vi "Axsun control.vi"() -> ()   [LabVIEW 2018]
uses:
  General/Controls/QueueNames.ctl
  General/Controls/Queue Manager Actions.ctl
  General/Controls/MessagePacket.ctl
  C:/Users/shuaibin/Documents/SerialSectOCT/SerialSectOCT/Software/Test Code/Stephan/Axsun Control/AxsunOCTControl.dll
  AxsunOCTControl.dll
panel:
  out "Cluster":cluster{i32, string[], string, dbl, string, i32}
  out "GUI error":errorcluster
  in  "Source current OFF":bool
  in  "Source current ON":bool
  in  "stop":bool
  in  "Laser OFF":bool
  in  "Laser ON":bool
  out "processor error":errorcluster
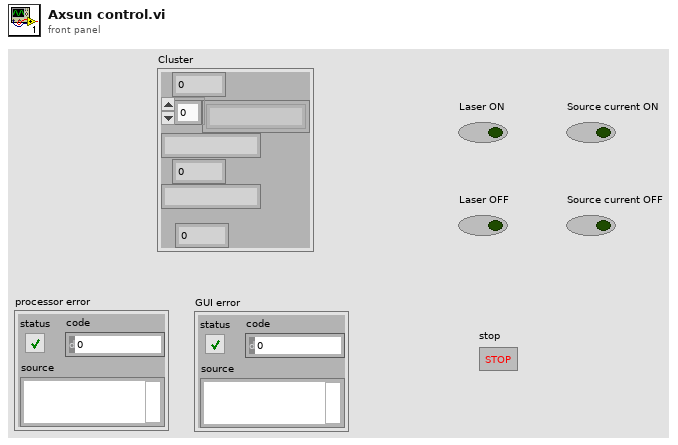
[diagram p1: front panel]
types:
  T1 = typedef "MessagePacket.ctl" = cluster{"Message":string, "Parameter":variant}
  T2 = typedef "Queue Manager Actions.ctl" = enum16{"Init", "Enqueue", "Enqueue All", "Preview Queue", "Dequeue", "Get Status", "Flush Queue", "Flush All Queues", "Release All Queues", "Release Queue", "Enqueue at Opposite End"}
  T3 = typedef "QueueNames.ctl" = enum16{"Main GUI", "Main Scan Processor", "Axsun GUI", "Axsun processor", "Main Display", "Main Table Stage GUI", "Main Table Stage Proc.", "Scan Engine", "Vibratome GUI", "Vibratome Processor", "Slice Engine"}
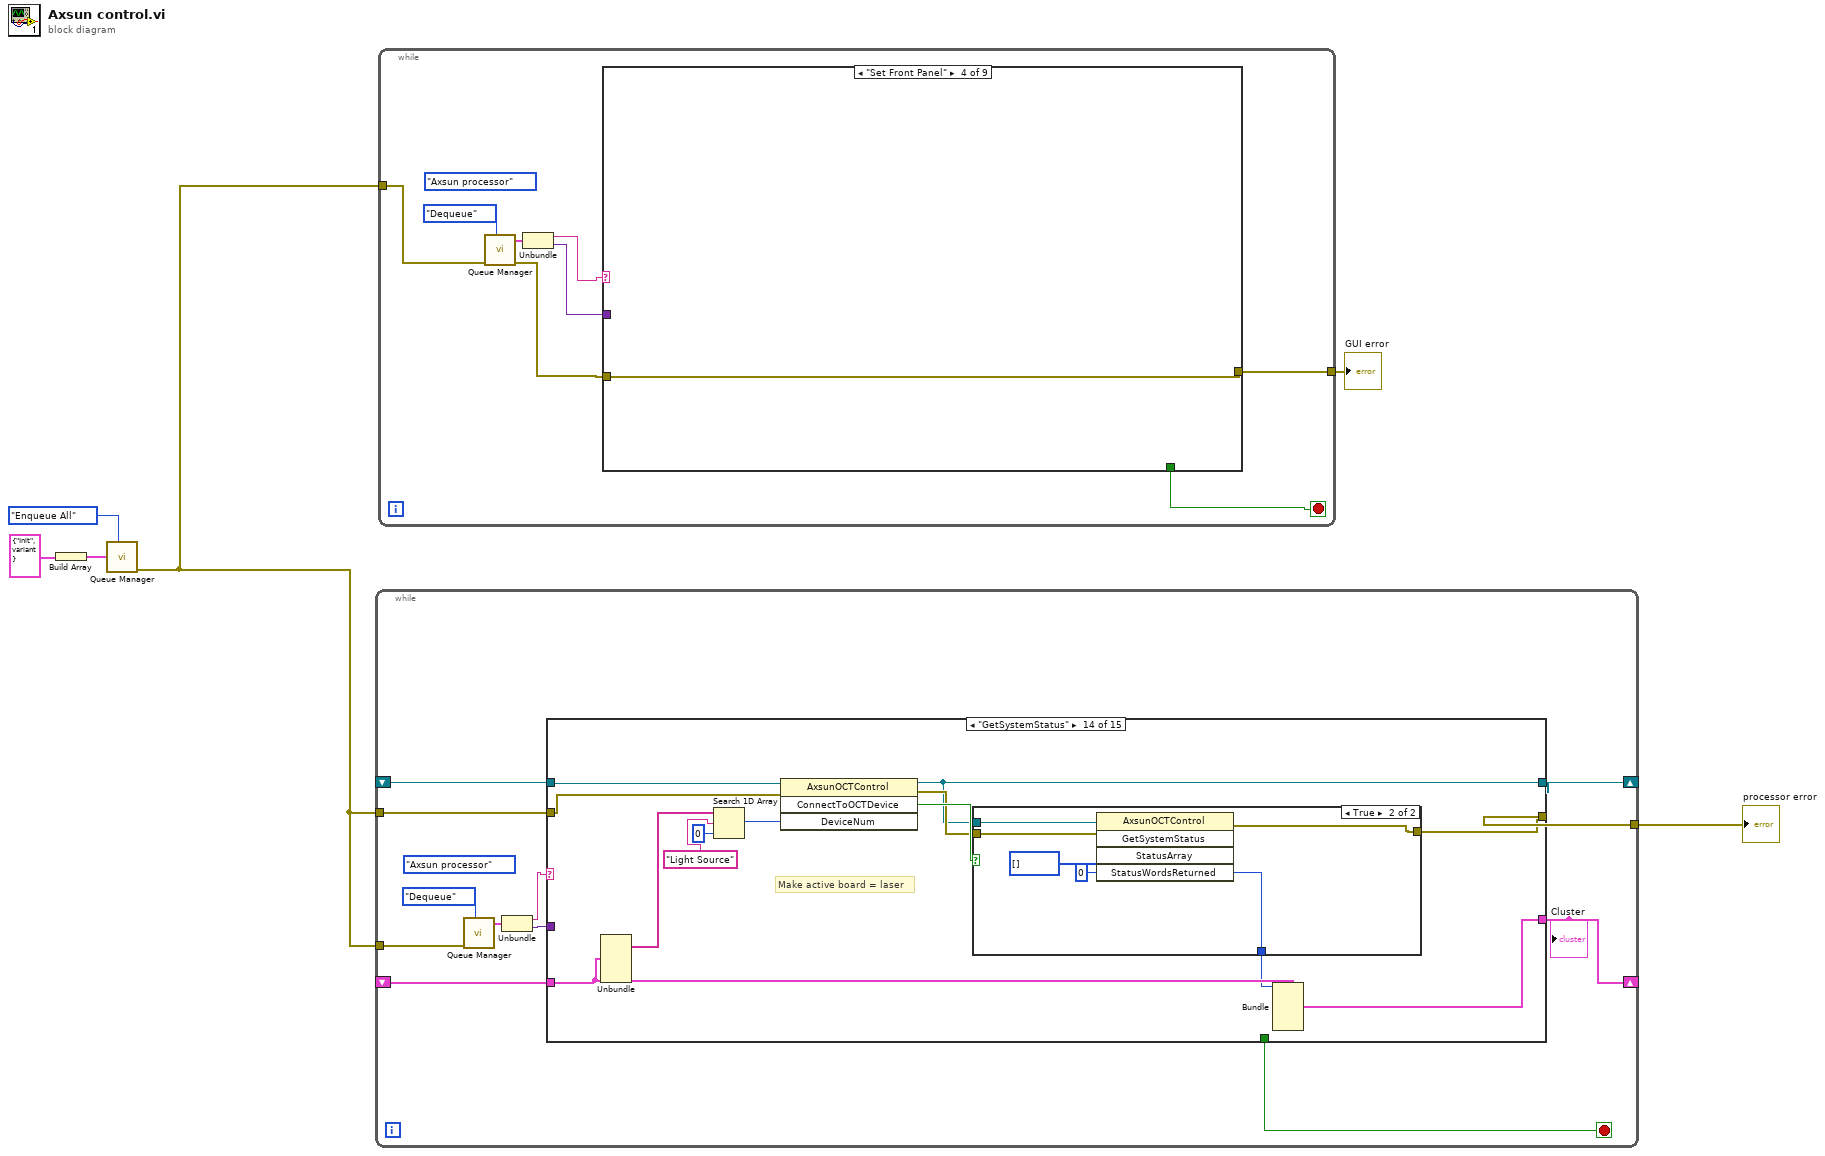
[diagram p0: block diagram]
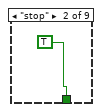
[diagram p3: hidden frame]
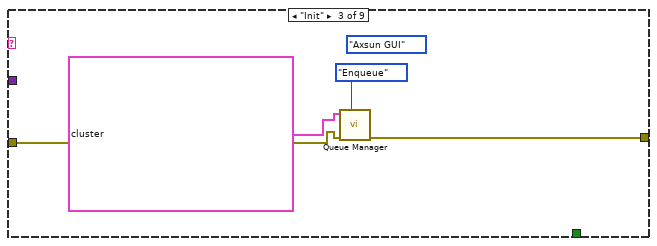
[diagram p4: hidden frame]
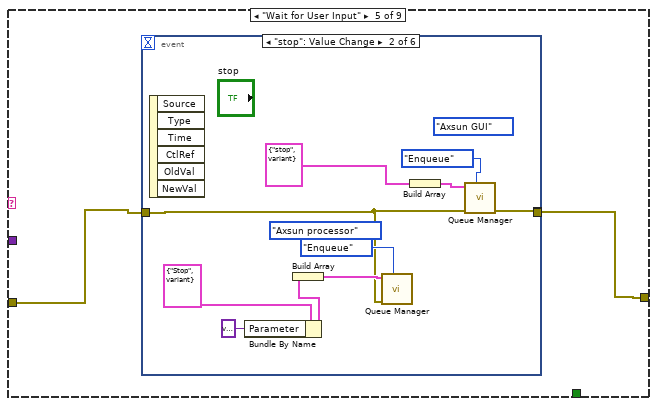
[diagram p5: hidden frame]
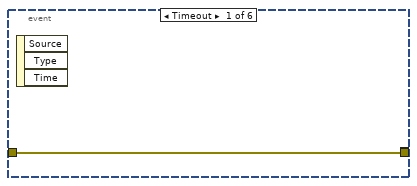
[diagram p6: hidden frame]
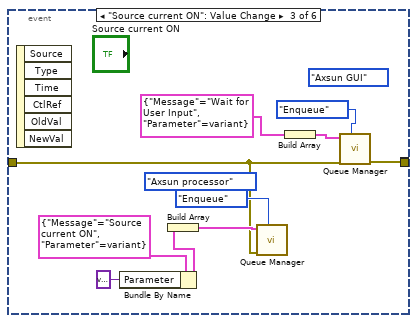
[diagram p7: hidden frame]
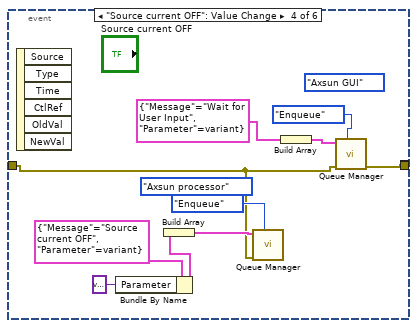
[diagram p8: hidden frame]
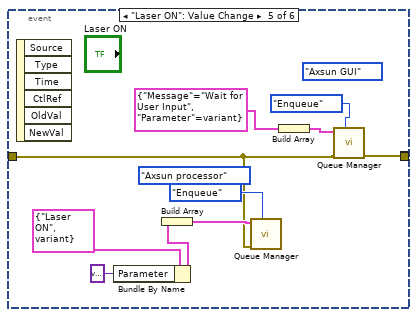
[diagram p9: hidden frame]
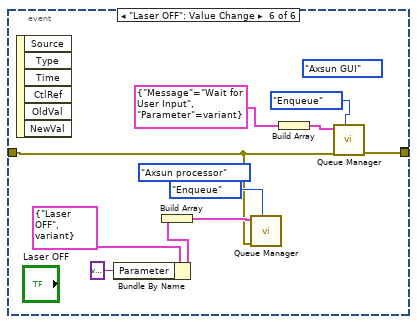
[diagram p10: hidden frame]
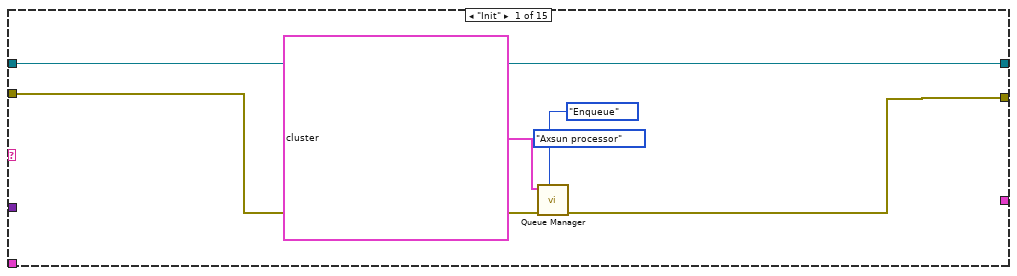
[diagram p15: hidden frame]
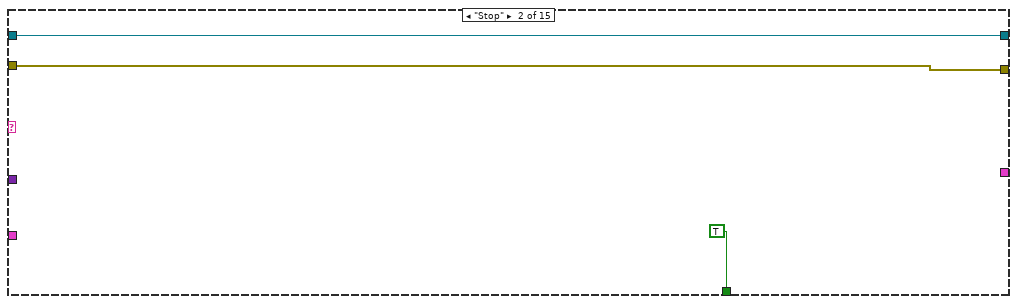
[diagram p16: hidden frame]
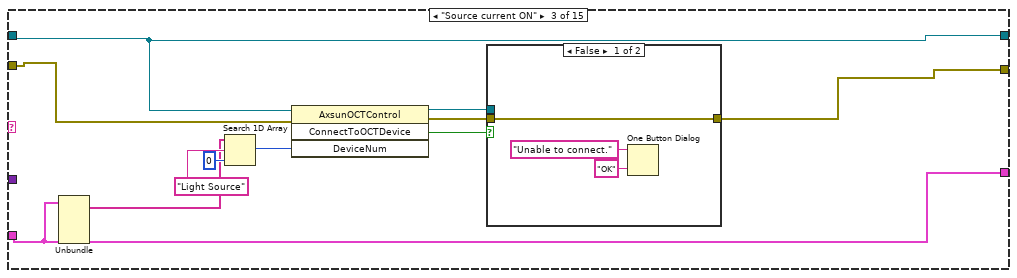
[diagram p17: hidden frame]
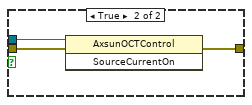
[diagram p18: hidden frame]
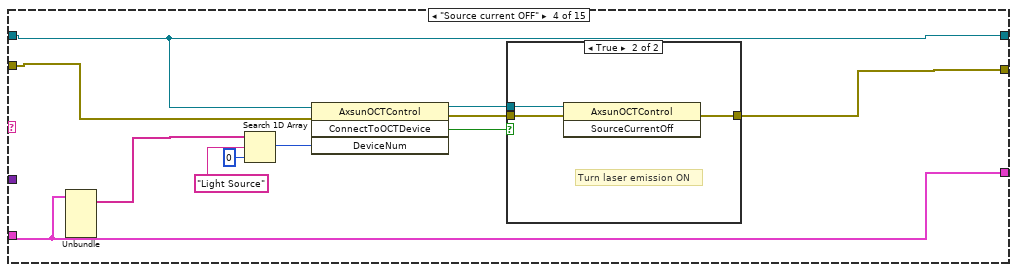
[diagram p19: hidden frame]
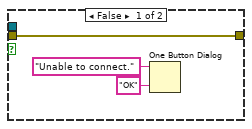
[diagram p20: hidden frame]
diagram:
  n1 = Build Array(T1 {"Message"="Init", "Parameter"=variant} ("Message Packet [In]")) -> (w4:T1[])
  n2 = call "Queue Manager.vi"("Action"=Queue_Manager_Actions."Enqueue All", "Message Packet Array"=w4) -> ("Error Out"=w2:errorcluster)  [unwired: 5 in, 4 out]
  n3 = while {
    shift-right: [w7] -> _
    shift-left: _ -> [w13]
    tunnel: w2 -> [w15]
    shift-right: [w8] -> _
    shift-left: _ -> [w11]
    tunnel: [w10] -> w3
    tunnel: w2 -> [w9]
    stop <- w14 stop-if-true
    (unwired) QueueNames."Axsun processor" ("Queue Name")
    n4 = call "Queue Manager.vi"("Action"=Queue_Manager_Actions."Dequeue", "Error In"=w9) -> ("Message Packet [Out]"=w17:T1)  [unwired: 5 in, 4 out]
    n5 = Unbundle(w17) -> ("Message"=w12:string, "Parameter"=w16:variant)
    n6 = case shown="\"GetSystemStatus\"" w12 {
      tunnel: w16 -> [_ _ _ _ _ _ _ _ _ _ _ _ _ _ _]
      tunnel: w15 -> [w23 w25 w31 w47 w63 w68 w84 w104 w122 w144 w163 w181 w188 w210 _]
      tunnel: [_ TRUE _ _ _ _ _ _ _ _ _ _ _ _ _] -> w14
      tunnel: w13 -> [w19 w24 w29 w46 w62 w69 w79 w102 w123 w142 w161 w182 w189 w211 _]
      tunnel: [w20 w25 w30 w48 w63 w66 w80 w103 w121 w143 w162 w180 w183 w205 w227] -> w10
      tunnel: [_ _ w28 w45 w61 w64 w77 w101 w119 w139 w160 w177 w184 w206 w226] -> w8
      tunnel: w11 -> [_ _ w28 w45 w61 w64 _ w101 w120 w141 w160 w178 w186 w208 w226]
      tunnel: [w19 w24 w29 w46 w62 w65 w79 w102 w123 w142 w161 w179 w189 w204 w228] -> w7
      frame "Init" {
        (unwired) QueueNames."Axsun processor" ("Queue Name")
        n7 = call "Queue Manager.vi"("Action"=Queue_Manager_Actions."Enqueue", "Error In"=w23, "Message Packet Array"=T1[] [{"Message"="Create handle", "Parameter"=variant}, {"Message"="Start Network Control Interface", "Parameter"=variant}, {"Message"="Get laser handle", "Parameter"=variant}, {"Message"="GetControlVersion", "Parameter"=variant}, {"Message"="GetSerialNum", "Parameter"=variant}, {"Message"="GetSystemStatus", "Parameter"=variant}, {"Message"="GetWaveLengthAtSweptTrigger", "Parameter"=variant}, {"Message"="GetLaserOnTime\nGetLaserOnTime", "Parameter"=variant}]) -> ("Error Out"=w20:errorcluster)  [unwired: 4 in, 4 out]
      }
      frame "Stop" {
      }
      frame "Source current ON" {
        n8 = Unbundle(w28) -> (w27:string[])  [unwired: 5 out]
        n9 = Search 1D Array(1D array=w27, element="Light Source", start index (0)=0) -> (index of element=w35:i32)
        n10 = invoke class="AxsunOCTControl" method="ConnectToOCTDevice"(reference=w29, error in=w31, "DeviceNum"=w35) -> (reference out=w34:refnum<k24>, error out=w33:errorcluster, "ConnectToOCTDevice"=w32:bool)  [unwired: 1 in, 1 out]
        n11 = case shown="False" w32 {
          tunnel: w34 -> [_ w43]
          tunnel: w33 -> [w40 w42]
          tunnel: [w40 w41] -> w30
          frame False {
            n12 = One Button Dialog(message="Unable to connect.", button name ("OK")="OK") -> ()  [unwired: 1 out]
          }
          frame True {
            n13 = invoke class="AxsunOCTControl" method="SourceCurrentOn"(reference=w43, error in=w42) -> (error out=w41:errorcluster)  [unwired: 1 in, 2 out]
          }
        }
      }
      frame "Source current OFF" {
        n14 = Unbundle(w45) -> (w44:string[])  [unwired: 5 out]
        n15 = Search 1D Array(1D array=w44, element="Light Source", start index (0)=0) -> (index of element=w52:i32)
        n16 = invoke class="AxsunOCTControl" method="ConnectToOCTDevice"(reference=w46, error in=w47, "DeviceNum"=w52) -> (reference out=w51:refnum<k24>, error out=w50:errorcluster, "ConnectToOCTDevice"=w49:bool)  [unwired: 1 in, 1 out]
        n17 = case shown="True" w49 {
          tunnel: w51 -> [_ w60]
          tunnel: w50 -> [w57 w59]
          tunnel: [w57 w58] -> w48
          frame False {
            n18 = One Button Dialog(message="Unable to connect.", button name ("OK")="OK") -> ()  [unwired: 1 out]
          }
          frame True {
            # "Turn laser emission ON"
            n19 = invoke class="AxsunOCTControl" method="SourceCurrentOff"(reference=w60, error in=w59) -> (error out=w58:errorcluster)  [unwired: 1 in, 2 out]
          }
        }
      }
      frame Default {
      }
      frame "Start Network Control Interface" {
        n20 = invoke class="AxsunOCTControl" method="StartNetworkControlInterface"(reference=w69, error in=w68) -> (reference out=w65:refnum<k24>, error out=w67:errorcluster)  [unwired: 1 in, 1 out]
        n21 = flat-sequence {
          tunnel: w67 -> [w70]
          tunnel: [w70] -> w66
          frame #0 {
            n22 = Wait (ms)(milliseconds to wait=2000) -> ()  [unwired: 1 out]
          }
        }
      }
      frame "Get laser handle" {
        n23 = invoke class="AxsunOCTControl" method="GetNumberOfOCTDevicesPresent"(reference=w79, error in=w84) -> (reference out=w83:refnum<k24>, error out=w81:errorcluster, "GetNumberOfOCTDevicesPresent"=w82:i32)  [unwired: 1 in]
        n24 = for {
          N: w82 -> [_]
          tunnel: w83 -> [w90]
          tunnel: w81 -> [w89]
          tunnel: [w85] -> w78 mode=indexing
          tunnel: [w87] -> w80
          tunnel: [w86] -> _ mode=indexing
          i -> [w88]
          n25 = invoke class="AxsunOCTControl" method="ConnectToOCTDevice"(reference=w90, error in=w89, "DeviceNum"=w88) -> (reference out=w94:refnum<k24>, error out=w93:errorcluster)  [unwired: 1 in, 2 out]
          n26 = stacked-sequence {
            tunnel: w94 -> [w99]
            tunnel: [w99] -> w92
            tunnel: w93 -> [w98]
            tunnel: [w98] -> w91
            frame #0 {
              n27 = Wait (ms)(milliseconds to wait=u32 20) -> ()  [unwired: 1 out]
            }
          }
          n28 = invoke class="AxsunOCTControl" method="GetSystemType"(reference=w92, error in=w91, "SystemType"=u32 0, "SystemTypeString"="") -> (reference out=w86:refnum<k24>, error out=w87:errorcluster, "SystemTypeString"=w85:string)  [unwired: 1 in, 2 out]
        }
        n29 = Bundle(0, w78, "GetControlVersion", 0.0, "", 0) -> (w77:cluster{i32, string[], string, dbl, string, i32})  [unwired: 1 in]
      }
      frame "Laser ON" {
        n30 = Unbundle(w101) -> (w100:string[])  [unwired: 5 out]
        n31 = Search 1D Array(1D array=w100, element="Light Source", start index (0)=0) -> (index of element=w108:i32)
        n32 = invoke class="AxsunOCTControl" method="ConnectToOCTDevice"(reference=w102, error in=w104, "DeviceNum"=w108) -> (reference out=w107:refnum<k24>, error out=w106:errorcluster, "ConnectToOCTDevice"=w105:bool)  [unwired: 1 in, 1 out]
        n33 = case shown="True" w105 {
          tunnel: w107 -> [_ w116]
          tunnel: w106 -> [w113 w115]
          tunnel: [w113 w114] -> w103
          frame False {
            n34 = One Button Dialog(message="Unable to .", button name ("OK")="OK") -> ()  [unwired: 1 out]
          }
          frame True {
            # "Turn laser emission ON"
            n35 = invoke class="AxsunOCTControl" method="StartScan"(reference=w116, error in=w115) -> (error out=w114:errorcluster)  [unwired: 1 in, 2 out]
          }
        }
      }
      frame "GetWaveLengthAtSweptTrigger" {
        n36 = Unbundle(w120) -> (w118:string[])  [unwired: 5 out]
        n37 = Search 1D Array(1D array=w118, element="Light Source", start index (0)=0) -> (index of element=w127:i32)
        n38 = invoke class="AxsunOCTControl" method="ConnectToOCTDevice"(reference=w123, error in=w122, "DeviceNum"=w127) -> (reference out=w126:refnum<k24>, error out=w125:errorcluster, "ConnectToOCTDevice"=w124:bool)  [unwired: 1 in, 1 out]
        n39 = case shown="False" w124 {
          tunnel: w126 -> [_ w137]
          tunnel: w125 -> [w132 w136]
          tunnel: [w132 w135] -> w121
          tunnel: [_ w133] -> w117
          frame False {
            n40 = One Button Dialog(message="Unable to .", button name ("OK")="OK") -> ()  [unwired: 1 out]
          }
          frame True {
            # "Turn laser emission ON"
            n41 = invoke class="AxsunOCTControl" method="GetWavelengthAtSweepTrigger"(reference=w137, error in=w136, "Wavelength"=0.0) -> (error out=w135:errorcluster, "Wavelength"=w133:dbl)  [unwired: 1 in, 2 out]
          }
        }
        n42 = Bundle(cluster=w120, w117) -> (w119:cluster{i32, string[], string, dbl, string, i32})  [unwired: 5 in]
      }
      frame "GetLaserOnTime" {
        # "Make active board = laser"
        n43 = Unbundle(w141) -> (w138:string[])  [unwired: 5 out]
        n44 = Search 1D Array(1D array=w138, element="Light Source", start index (0)=0) -> (index of element=w150:i32)
        n45 = invoke class="AxsunOCTControl" method="ConnectToOCTDevice"(reference=w142, error in=w144, "DeviceNum"=w150) -> (reference out=w146:refnum<k24>, error out=w147:errorcluster, "ConnectToOCTDevice"=w145:bool)  [unwired: 1 in, 1 out]
        n46 = case shown="False" w145 {
          tunnel: w147 -> [w153 w157]
          tunnel: w146 -> [_ w158]
          tunnel: [w153 w156] -> w143
          tunnel: [_ w154] -> w140
          frame False {
            n47 = One Button Dialog(message="Unable to connect.", button name ("OK")="OK") -> ()  [unwired: 1 out]
          }
          frame True {
            n48 = invoke class="AxsunOCTControl" method="GetLaserOnTime"(reference=w158, error in=w157, "LaserOnTimeSeconds"=u32 0) -> (error out=w156:errorcluster, "LaserOnTimeSeconds"=w154:u32)  [unwired: 1 in, 2 out]
          }
        }
        n49 = Bundle(cluster=w141, w140) -> (w139:cluster{i32, string[], string, dbl, string, i32})  [unwired: 5 in]
      }
      frame "Laser OFF" {
        # "Make active board = laser"
        n50 = Unbundle(w160) -> (w159:string[])  [unwired: 5 out]
        n51 = Search 1D Array(1D array=w159, element="Light Source", start index (0)=0) -> (index of element=w167:i32)
        n52 = invoke class="AxsunOCTControl" method="ConnectToOCTDevice"(reference=w161, error in=w163, "DeviceNum"=w167) -> (reference out=w166:refnum<k24>, error out=w165:errorcluster, "ConnectToOCTDevice"=w164:bool)  [unwired: 1 in, 1 out]
        n53 = case shown="True" w164 {
          tunnel: w166 -> [_ w175]
          tunnel: w165 -> [w172 w174]
          tunnel: [w172 w173] -> w162
          frame False {
            n54 = One Button Dialog(message="Unable to connect.", button name ("OK")="OK") -> ()  [unwired: 1 out]
          }
          frame True {
            # "Turn laser emission ON"
            n55 = invoke class="AxsunOCTControl" method="StopScan"(reference=w175, error in=w174) -> (error out=w173:errorcluster)  [unwired: 1 in, 2 out]
          }
        }
      }
      frame "GetControlVersion" {
        n56 = invoke class="AxsunOCTControl" method="GetControlVersion"(reference=w182, error in=w181) -> (reference out=w179:refnum<k24>, error out=w180:errorcluster, "GetControlVersion"=w176:string)  [unwired: 1 in]
        n57 = Bundle(cluster=w178, w176) -> (w177:cluster{i32, string[], string, dbl, string, i32})  [unwired: 5 in]
      }
      frame "GetSerialNum" {
        n58 = Unbundle(w186) -> (w187:string[])  [unwired: 5 out]
        n59 = Search 1D Array(1D array=w187, element="Light Source", start index (0)=0) -> (index of element=w193:i32)
        n60 = invoke class="AxsunOCTControl" method="ConnectToOCTDevice"(reference=w189, error in=w188, "DeviceNum"=w193) -> (reference out=w192:refnum<k24>, error out=w191:errorcluster, "ConnectToOCTDevice"=w190:bool)  [unwired: 1 in, 1 out]
        n61 = case shown="True" w190 {
          tunnel: w192 -> [_ w203]
          tunnel: w191 -> [w198 w202]
          tunnel: [w198 w201] -> w183
          tunnel: [_ w199] -> w185
          frame False {
            n62 = One Button Dialog(message="Unable to connect.", button name ("OK")="OK") -> ()  [unwired: 1 out]
          }
          frame True {
            n63 = invoke class="AxsunOCTControl" method="GetSerialNum"(reference=w203, error in=w202, "SerialNum"="") -> (error out=w201:errorcluster, "SerialNum"=w199:string)  [unwired: 1 in, 2 out]
          }
        }
        n64 = Bundle(cluster=w186, w185) -> (w184:cluster{i32, string[], string, dbl, string, i32})  [unwired: 5 in]
      }
      frame "GetSystemStatus" {
        # "Make active board = laser"
        n65 = Unbundle(w208) -> (w209:string[])  [unwired: 5 out]
        n66 = Search 1D Array(1D array=w209, element="Light Source", start index (0)=0) -> (index of element=w216:i32)
        n67 = invoke class="AxsunOCTControl" method="ConnectToOCTDevice"(reference=w211, error in=w210, "DeviceNum"=w216) -> (reference out=w204:refnum<k24>, error out=w212:errorcluster, "ConnectToOCTDevice"=w213:bool)  [unwired: 1 in, 1 out]
        n68 = case shown="True" w213 {
          tunnel: w212 -> [w219 w224]
          tunnel: w204 -> [_ w225]
          tunnel: [w219 w221] -> w205
          tunnel: [_ w220] -> w207
          frame False {
            n69 = One Button Dialog(message="Unable to connect.", button name ("OK")="OK") -> ()  [unwired: 1 out]
          }
          frame True {
            n70 = invoke class="AxsunOCTControl" method="GetSystemStatus"(reference=w225, error in=w224, "StatusArray"=u32[] [], "StatusWordsReturned"=u32 0) -> (error out=w221:errorcluster, "StatusWordsReturned"=w220:u32)  [unwired: 1 in, 3 out]
          }
        }
        n71 = Bundle(cluster=w208, w207) -> (w206:cluster{i32, string[], string, dbl, string, i32})  [unwired: 5 in]
      }
      frame "Create handle" {
        n72 = constructor class="AxsunOCTControl"() -> (reference out=w228:refnum<k24>, error out=w227:errorcluster)  [unwired: 3 in, 1 out]
      }
    }
    "Cluster" <- w8
  }
  "processor error" <- w3
  n73 = while {
    tunnel: w2 -> [w234]
    tunnel: [w230] -> w1
    stop <- w229 stop-if-true
    (unwired) QueueNames."Axsun processor" ("Queue Name")
    n74 = call "Queue Manager.vi"("Action"=Queue_Manager_Actions."Dequeue", "Error In"=w234) -> ("Error Out"=w231:errorcluster, "Message Packet [Out]"=w235:T1)  [unwired: 5 in, 3 out]
    n75 = Unbundle(w235) -> ("Message"=w233:string, "Parameter"=w232:variant)
    n76 = case shown="\"Set Front Panel\"" w233 {
      tunnel: w232 -> [_ _ _ _ _ _ _ _ _]
      tunnel: w231 -> [w237 _ w242 w243 w245 w297 w298 w299 w300]
      tunnel: [w237 _ w240 w243 w244 w297 w298 w299 w300] -> w230
      tunnel: [_ TRUE _ _ _ _ _ _ _] -> w229
      frame "False", Default {
      }
      frame "stop" {
      }
      frame "Init" {
        (unwired) QueueNames."Axsun GUI" ("Queue Name")
        n77 = call "Queue Manager.vi"("Action"=Queue_Manager_Actions."Enqueue", "Error In"=w242, "Message Packet Array"=T1[] [{"Message"="Wait for Complete", "Parameter"=variant}, {"Message"="Set Front Panel", "Parameter"=variant}, {"Message"="Load User Settings", "Parameter"=variant}, {"Message"="Configure Hardware", "Parameter"=variant}, {"Message"="Configure Hardware", "Parameter"=variant}, {"Message"="Wait for User Input", "Parameter"=variant}]) -> ("Error Out"=w240:errorcluster)  [unwired: 4 in, 4 out]
      }
      frame "Set Front Panel" {
      }
      frame "Wait for User Input" {
        n78 = event shown="[1] \"stop\": Value Change" {
          selector: _ -> [_ _ _ _ _ _]
          dyn-events: _ -> [_ _ _ _ _ _]
          timeout: _ -> [_ _ _ _ _ _]
          tunnel: w245 -> [w246 w247 w257 w267 w277 w287]
          tunnel: [_ w248 w258 w268 w281 w289] -> w244
          tunnel: [w246 _ _ _ _ _] -> _
          event Timeout {
            n79 = event-data() -> ()  [unwired: 1 in, 3 out]
          }
          event "stop": Value Change {
            (unwired) QueueNames."Axsun processor" ("Queue Name")
            (unwired) QueueNames."Axsun GUI" ("Queue Name")
            n80 = event-data() -> ()  [unwired: 1 in, 6 out]
            n81 = Bundle By Name(cluster=T1 {"Message"="Stop", "Parameter"=variant} ("Message Packet [In]"), "Parameter"=variant) -> (w253:T1)
            n82 = Build Array(w253) -> (w251:T1[])
            n83 = call "Queue Manager.vi"("Action"=Queue_Manager_Actions."Enqueue", "Error In"=w247, "Message Packet Array"=w251) -> ()  [unwired: 4 in, 5 out]
            n84 = Build Array(T1 {"Message"="stop", "Parameter"=variant} ("Message Packet [In]")) -> (w256:T1[])
            n85 = call "Queue Manager.vi"("Action"=Queue_Manager_Actions."Enqueue", "Error In"=w247, "Message Packet Array"=w256) -> ("Error Out"=w248:errorcluster)  [unwired: 4 in, 4 out]
          }
          event "Source current ON": Value Change {
            (unwired) QueueNames."Axsun processor" ("Queue Name")
            (unwired) QueueNames."Axsun GUI" ("Queue Name")
            n86 = event-data() -> ()  [unwired: 1 in, 6 out]
            n87 = Bundle By Name(cluster=T1 {"Message"="Source current ON", "Parameter"=variant} ("Message Packet [In]"), "Parameter"=variant) -> (w263:T1)
            n88 = Build Array(w263) -> (w261:T1[])
            n89 = call "Queue Manager.vi"("Action"=Queue_Manager_Actions."Enqueue", "Error In"=w257, "Message Packet Array"=w261) -> ()  [unwired: 4 in, 5 out]
            n90 = Build Array(T1 {"Message"="Wait for User Input", "Parameter"=variant} ("Message Packet [In]")) -> (w266:T1[])
            n91 = call "Queue Manager.vi"("Action"=Queue_Manager_Actions."Enqueue", "Error In"=w257, "Message Packet Array"=w266) -> ("Error Out"=w258:errorcluster)  [unwired: 4 in, 4 out]
          }
          event "Source current OFF": Value Change {
            (unwired) QueueNames."Axsun processor" ("Queue Name")
            (unwired) QueueNames."Axsun GUI" ("Queue Name")
            n92 = event-data() -> ()  [unwired: 1 in, 6 out]
            n93 = Bundle By Name(cluster=T1 {"Message"="Source current OFF", "Parameter"=variant} ("Message Packet [In]"), "Parameter"=variant) -> (w273:T1)
            n94 = Build Array(w273) -> (w271:T1[])
            n95 = call "Queue Manager.vi"("Action"=Queue_Manager_Actions."Enqueue", "Error In"=w267, "Message Packet Array"=w271) -> ()  [unwired: 4 in, 5 out]
            n96 = Build Array(T1 {"Message"="Wait for User Input", "Parameter"=variant} ("Message Packet [In]")) -> (w276:T1[])
            n97 = call "Queue Manager.vi"("Action"=Queue_Manager_Actions."Enqueue", "Error In"=w267, "Message Packet Array"=w276) -> ("Error Out"=w268:errorcluster)  [unwired: 4 in, 4 out]
          }
          event "Laser ON": Value Change {
            (unwired) QueueNames."Axsun processor" ("Queue Name")
            (unwired) QueueNames."Axsun GUI" ("Queue Name")
            n98 = event-data() -> ()  [unwired: 1 in, 6 out]
            n99 = Bundle By Name(cluster=T1 {"Message"="Laser ON", "Parameter"=variant} ("Message Packet [In]"), "Parameter"=variant) -> (w283:T1)
            n100 = Build Array(w283) -> (w280:T1[])
            n101 = call "Queue Manager.vi"("Action"=Queue_Manager_Actions."Enqueue", "Error In"=w277, "Message Packet Array"=w280) -> ()  [unwired: 4 in, 5 out]
            n102 = Build Array(T1 {"Message"="Wait for User Input", "Parameter"=variant} ("Message Packet [In]")) -> (w286:T1[])
            n103 = call "Queue Manager.vi"("Action"=Queue_Manager_Actions."Enqueue", "Error In"=w277, "Message Packet Array"=w286) -> ("Error Out"=w281:errorcluster)  [unwired: 4 in, 4 out]
          }
          event "Laser OFF": Value Change {
            (unwired) QueueNames."Axsun processor" ("Queue Name")
            (unwired) QueueNames."Axsun GUI" ("Queue Name")
            n104 = event-data() -> ()  [unwired: 1 in, 6 out]
            n105 = Bundle By Name(cluster=T1 {"Message"="Laser OFF", "Parameter"=variant} ("Message Packet [In]"), "Parameter"=variant) -> (w293:T1)
            n106 = Build Array(w293) -> (w291:T1[])
            n107 = call "Queue Manager.vi"("Action"=Queue_Manager_Actions."Enqueue", "Error In"=w287, "Message Packet Array"=w291) -> ()  [unwired: 4 in, 5 out]
            n108 = Build Array(T1 {"Message"="Wait for User Input", "Parameter"=variant} ("Message Packet [In]")) -> (w296:T1[])
            n109 = call "Queue Manager.vi"("Action"=Queue_Manager_Actions."Enqueue", "Error In"=w287, "Message Packet Array"=w296) -> ("Error Out"=w289:errorcluster)  [unwired: 4 in, 4 out]
          }
        }
      }
      frame "Wait for Complete" {
      }
      frame "Configure Hardware" {
      }
      frame "Load User Settings" {
      }
      frame "Init Variables" {
      }
    }
  }
  "GUI error" <- w1
